vi "Acoustic Functional Test.vi"(0 "TSM context":T2, 5 "Limits File Path":path, 7 "Write to Limit File?":bool) -> (4 "Results":T1[](array[typedef]) {"Site Num" format="Site %#_g"}, 15 "error out":errorcluster)   [LabVIEW 2020]
doc: "Performs Functional test by sweeping over various frequency logarithmically over a single amplitude and getting the equivalent dB SPL. This Obtained dB SPL is compared with Limits files to validate \"In Range?\" functionality."
uses:
  <vilib>/NI_TestStand_SemiconductorModule/NI_TestStand_Semiconductor_Module.lvlibp/PinMap/General/SemiconductorModuleContext.ctl
  SubVIs/Site Info.ctl
  Common/Utility/Calibration Sweep/Sweep Parameters.ctl
  Limits File APIs/Plot Data.ctl
  <vilib>/NI_TestStand_SemiconductorModule/NI_TestStand_Semiconductor_Module.lvlibp
panel:
  in  "Exit":bool
  out "dBSPL Frequency Graph":cluster{"Frequency(Hz)":dbl[], "dB SPL":dbl[]}[](graph)
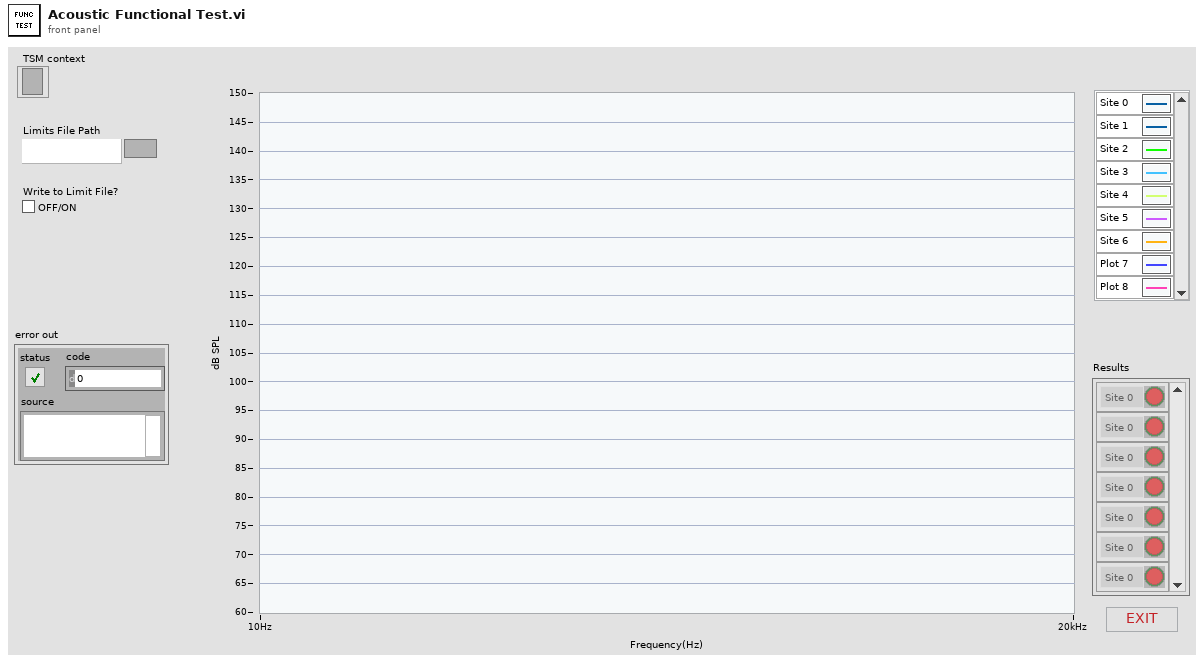
[diagram p1: front panel]
types:
  T1 = typedef "Site Info.ctl" = cluster{"Site Num":i32, "In Range?":bool}
  T2 = typedef "NI_TestStand_Semiconductor_Module.lvlibp/SemiconductorModuleContext.ctl" = refnum<k7>
  T3 = typedef "Sweep Parameters.ctl" = cluster{"Start":dbl, "End":dbl, "Samples":i32}
  T4 = typedef "Plot Data.ctl" = cluster{"Frequency(Hz)":dbl[], "dB SPL":dbl[]}
  T5 = cluster{"TSM context":T2, "Site Numbers":i32[], "Limits File Path":path, "Speaker Samp Rate (Hz)":dbl, "Ref Mic Samp Rate (Hz)":dbl, "Amplitude (V)":dbl, "Coarse Freq Sweep (Hz)":T3, "Fine Freq Sweep (Hz)":T3, "Positive Limit Plot":T4, "Negative Limit Plot":T4, "Graph Data":T4[], "Graph Ref":refnum<vi>, "Write Limit File?":bool, "Per-Site In Range?":T1[]}
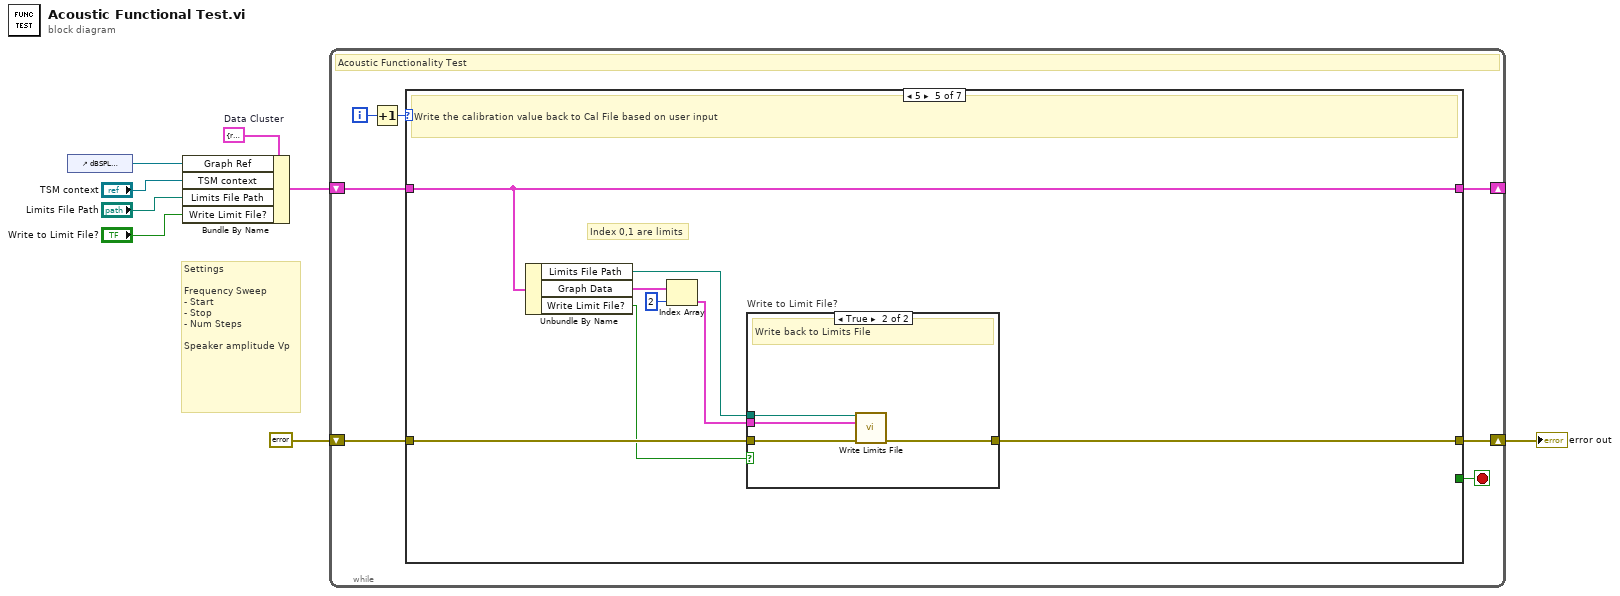
[diagram p0: block diagram]
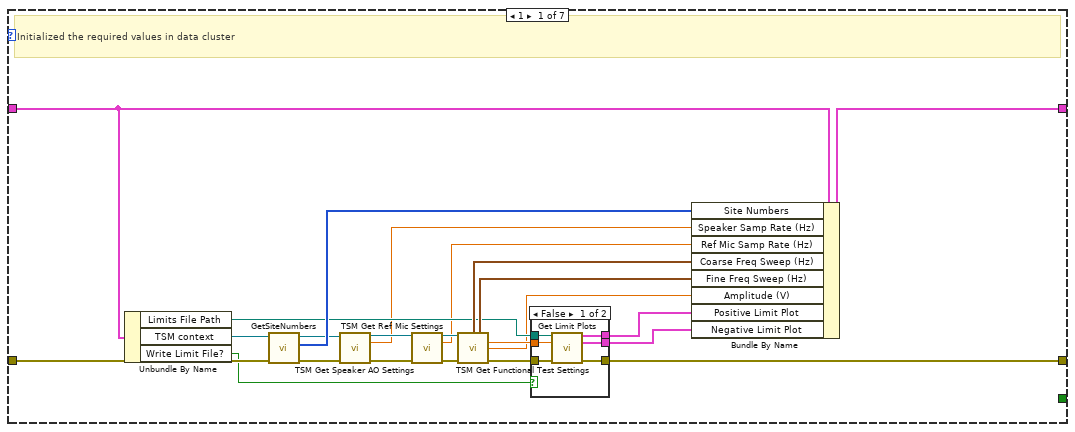
[diagram p2: hidden frame]
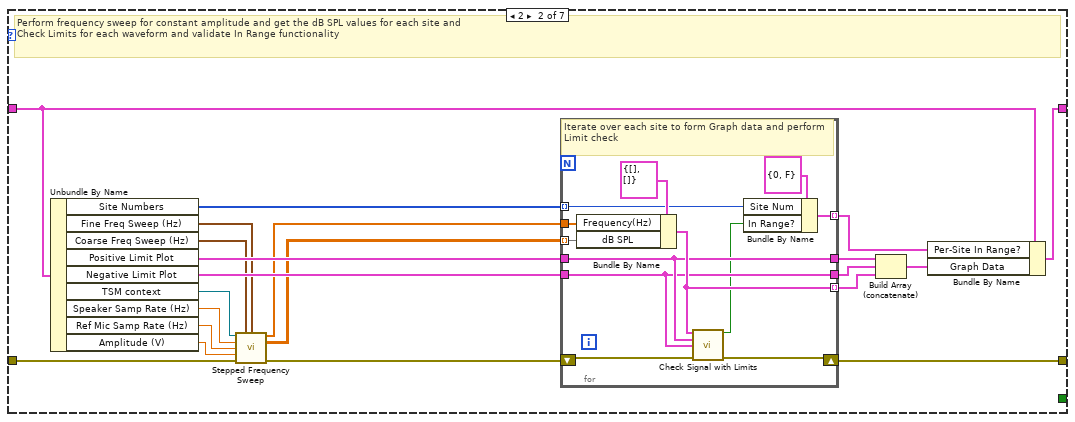
[diagram p4: hidden frame]
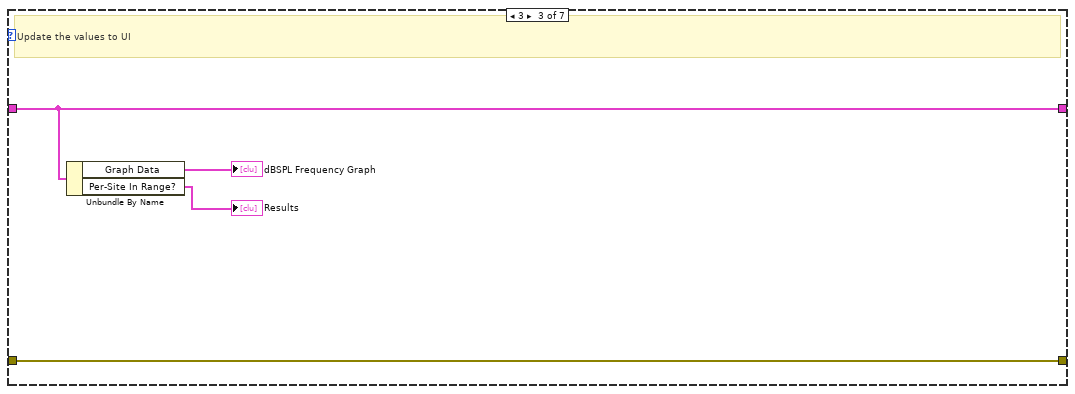
[diagram p5: hidden frame]
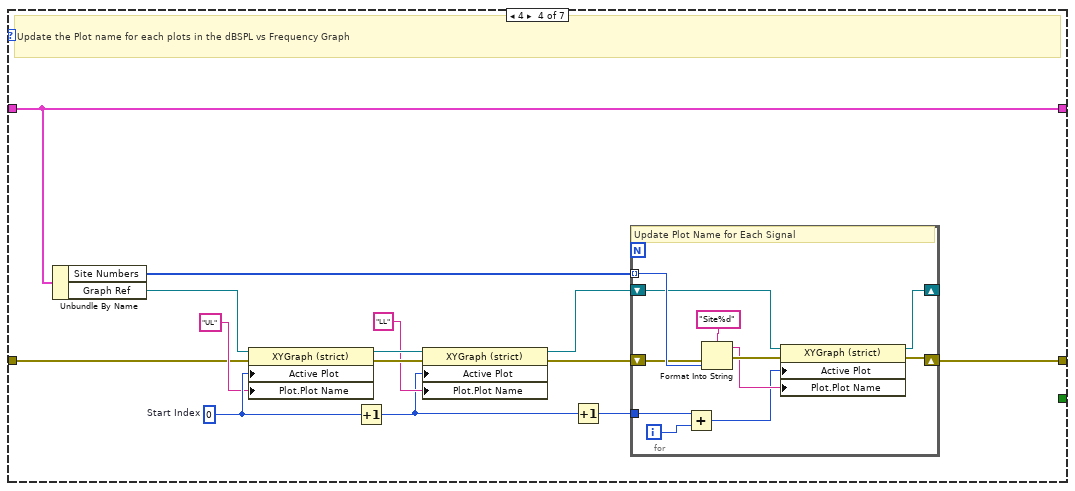
[diagram p6: hidden frame]
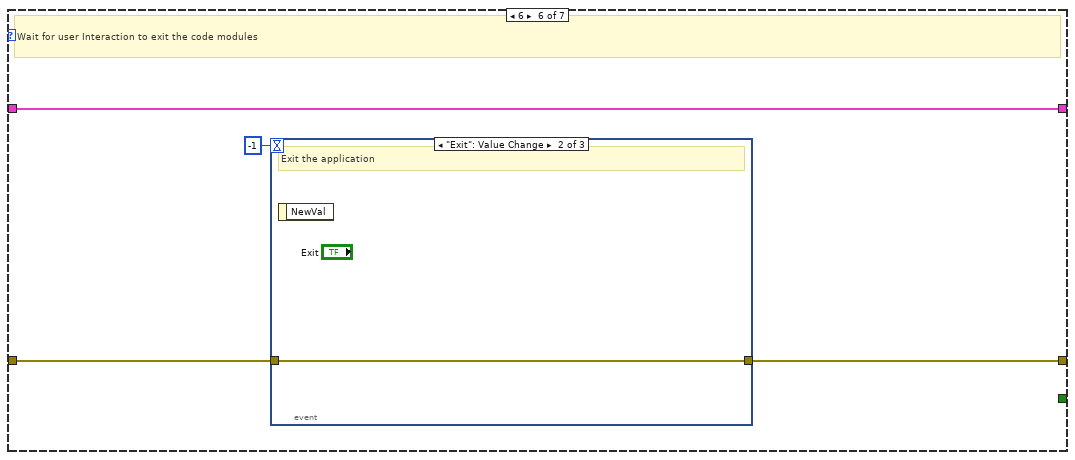
[diagram p8: hidden frame]
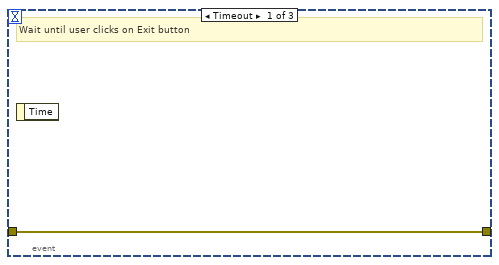
[diagram p9: hidden frame]
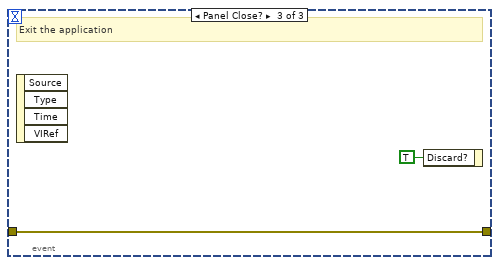
[diagram p10: hidden frame]
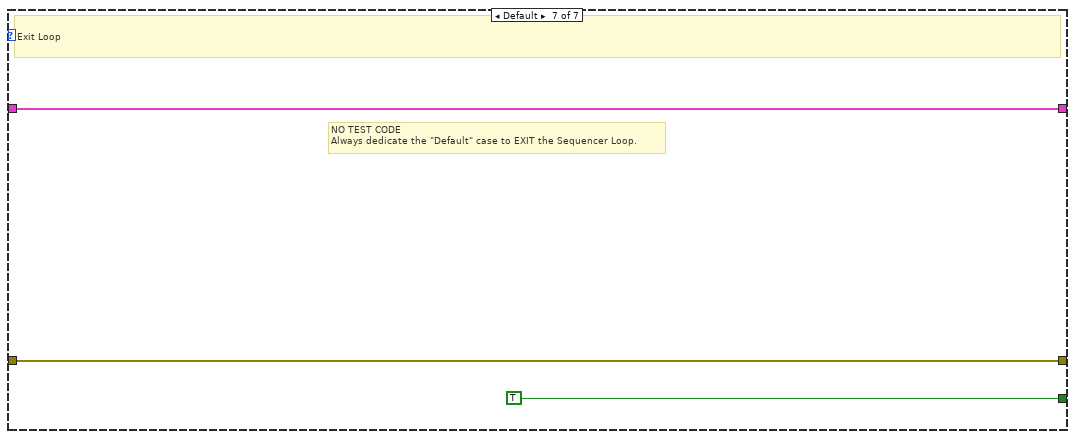
[diagram p11: hidden frame]
diagram:
  w6 = T5 {"TSM context"=refnum, "Site Numbers"=[], "Limits File Path"=path "", "Speaker Samp Rate (Hz)"=0.0, "Ref Mic Samp Rate (Hz)"=0.0, "Amplitude (V)"=0.0, "Coarse Freq Sweep (Hz)"={"Start"=0.0, "End"=0.0, "Samples"=0}, "Fine Freq Sweep (Hz)"={"Start"=0.0, "End"=0.0, "Samples"=0}, "Positive Limit Plot"={"Frequency(Hz)"=[], "dB SPL"=[]}, "Negative Limit Plot"={"Frequency(Hz)"=[], "dB SPL"=[]}, "Graph Data"=[], "Graph Ref"=refnum, "Write Limit File?"=FALSE, "Per-Site In Range?"=[]}  # Data Cluster
  # "Settings\n\nFrequency Sweep\n- Start\n- Stop\n- Num Steps\n\nSpeaker amplitude Vp"
  n1 = control-ref of="dBSPL Frequency Graph"() -> (w3:refnum<vi>)
  n2 = Bundle By Name(cluster=w6, "Graph Ref"=w3, "TSM context"="TSM context", "Limits File Path"="Limits File Path", "Write Limit File?"="Write to Limit File?") -> (w5:T5)
  n3 = while {
    shift-right: [w13] -> w8
    shift-left: errorcluster {"status"=FALSE, "code"=0, "source"=""} ("error in") -> [w14]
    shift-right: [w9] -> _
    shift-left: w5 -> [w10]
    i -> [w15]
    stop <- w11 stop-if-true
    # "Acoustic Functionality Test"
    n4 = Increment(x=w15) -> (x+1=w12:i32)
    n5 = case shown="5" w12 {
      tunnel: [w28 w63 w82 w83 w110 w122 w130] -> w13
      tunnel: w14 -> [w38 w57 w82 w89 w111 w123 w130]
      tunnel: [_ _ _ _ _ _ TRUE] -> w11
      tunnel: w10 -> [w35 w66 w81 w96 w115 w124 w129]
      tunnel: [w37 w62 w81 w96 w115 w124 w129] -> w9
      frame 1 {
        # "Initialized the required values in data cluster"
        n6 = Unbundle By Name(w35) -> ("Limits File Path"=w29:path, "TSM context"=w34:T2, "Write Limit File?"=w17:bool)
        n7 = call <vilib>:"GetSiteNumbers.vi"("error in (no error)"=w38, "Semiconductor Module Context"=w34) -> ("error out"=w23:errorcluster, "Site Numbers"=w36:i32[], "Semiconductor Module Context Out"=w22:T2)  [unwired: 6 in, 1 out]
        n8 = call "TSM Get Speaker AO Settings.vi"("TSM context"=w22, "error in (no error)"=w23) -> ("TSM context Out"=w21:T2, "Sampling Rate (Hz)"=w19:dbl, "error out"=w18:errorcluster)  [unwired: 9 in, 2 out]
        n9 = call "TSM Get Ref Mic Settings.vi"("TSM context"=w21, "error in (no error)"=w18) -> ("TSM context Out"=w24:T2, "Sampling Rate (Hz)"=w20:dbl, "error out"=w25:errorcluster)  [unwired: 8 in, 3 out]
        n10 = call "TSM Get Functional Test Settings.vi"("TSM context"=w24, "error in (no error)"=w25) -> ("Coarse Freq Sweep (Hz)"=w33:T3, "Fine Freq Sweep (Hz)"=w32:T3, "Limit (dB SPL)"=w30:dbl, "Speaker Amplitude (V)"=w16:dbl, "error out"=w31:errorcluster)  [unwired: 8 in, 1 out]
        n11 = case shown="False" w17 {
          tunnel: w31 -> [w44 w45]
          tunnel: w30 -> [w43 _]
          tunnel: w29 -> [w42 _]
          tunnel: [w41 w45] -> w28
          tunnel: [w40 _] -> w27
          tunnel: [w39 _] -> w26
          frame False {
            n12 = call "Get Limit Plots.vi"("Limits File Path"=w42, "Limit Range (dB SPL)"=w43, "error in (no error)"=w44) -> ("Positive Limit Plot"=w40:T4, "Negative Limit Plot"=w39:T4, "error out"=w41:errorcluster)  [unwired: 10 in]
          }
          frame True {
          }
        }
        n13 = Bundle By Name(cluster=w35, "Site Numbers"=w36, "Speaker Samp Rate (Hz)"=w19, "Ref Mic Samp Rate (Hz)"=w20, "Coarse Freq Sweep (Hz)"=w33, "Fine Freq Sweep (Hz)"=w32, "Amplitude (V)"=w16, "Positive Limit Plot"=w27, "Negative Limit Plot"=w26) -> (w37:T5)
      }
      frame 2 {
        # "Perform frequency sweep for constant amplitude and get the dB SPL values for each site and\nCheck Limits for each waveform and validate In Range functionality"
        n14 = Unbundle By Name(w66) -> ("Site Numbers"=w49:i32[], "Fine Freq Sweep (Hz)"=w54:T3, "Coarse Freq Sweep (Hz)"=w55:T3, "Positive Limit Plot"=w65:T4, "Negative Limit Plot"=w64:T4, "TSM context"=w53:T2, "Speaker Samp Rate (Hz)"=w52:dbl, "Ref Mic Samp Rate (Hz)"=w47:dbl, "Amplitude (V)"=w46:dbl)
        n15 = call "Stepped Frequency Sweep.vi"("Semiconductor Module Context"=w53, "Coarse Frequency Sweep (Hz)"=w55, "Fine Frequency Sweep (Hz)"=w54, "Speaker Sampling Rate (Hz)"=w52, "Ref Mic Sampling Rate (Hz)"=w47, "Amplitude (V)"=w46, "error in (no error)"=w57) -> ("Frequency (Hz)"=w51:dbl[], "Per-Site Per-Frequency dbSPL"=w50:dbl[][], "error out"=w56:errorcluster)  [unwired: 6 in]
        n16 = for {
          tunnel: [w73] -> w58 mode=indexing
          tunnel: w51 -> [w78]
          tunnel: w50 -> [w77] mode=indexing
          tunnel: w65 -> [w72]
          shift-right: [w74] -> w63
          shift-left: w56 -> [w75]
          tunnel: w64 -> [w71]
          tunnel: [w72] -> w61
          tunnel: [w71] -> w60
          tunnel: w49 -> [w69] mode=indexing
          tunnel: [w67] -> w48 mode=indexing
          # "Iterate over each site to form Graph data and perform Limit check"
          n17 = Bundle By Name(cluster=T4 {"Frequency(Hz)"=[], "dB SPL"=[]} ("Plot Data"), "Frequency(Hz)"=w78, "dB SPL"=w77) -> (w73:T4)
          n18 = call "Check Signal with Limits.vi"("Signal"=w73, "Positive Limit"=w72, "Negative Limit"=w71, "error in (no error)"=w75) -> ("In Range?"=w68:bool, "error out"=w74:errorcluster)  [unwired: 10 in]
          n19 = Bundle By Name(cluster=T1 {"Site Num"=0, "In Range?"=FALSE} ("Site Info"), "Site Num"=w69, "In Range?"=w68) -> (w67:T1)
        }
        n20 = Build Array (concatenate)(w61, w60, w58) -> (w59:T4[])
        n21 = Bundle By Name(cluster=w66, "Per-Site In Range?"=w48, "Graph Data"=w59) -> (w62:T5)
      }
      frame 3 {
        # "Update the values to UI"
        n22 = Unbundle By Name(w81) -> ("Graph Data"=→"dBSPL Frequency Graph":T4[], "Per-Site In Range?"=→"Results":T1[])
      }
      frame 4 {
        w94 = 0  # Start Index
        # "Update the Plot name for each plots in the dBSPL vs Frequency Graph"
        n23 = Unbundle By Name(w96) -> ("Site Numbers"=w95:i32[], "Graph Ref"=w87:refnum<vi>)
        n24 = property on="Property Node" class="XYGraph (strict)"(reference=w87, error in=w89, "Active Plot"=w94, "Plot.Plot Name"="UL" ("format string")) -> (reference out=w92:refnum<vi>, error out=w93:errorcluster)
        n25 = Increment(x=w94) -> (x+1=w85:i32)
        n26 = property on="Property Node" class="XYGraph (strict)"(reference=w92, error in=w93, "Active Plot"=w85, "Plot.Plot Name"="LL" ("format string")) -> (reference out=w86:refnum<vi>, error out=w88:errorcluster)
        n27 = Increment(x=w85) -> (x+1=w84:i32)
        n28 = for {
          shift-right: [w104] -> w83
          shift-left: w88 -> [w102]
          tunnel: w95 -> [w103] mode=indexing
          shift-right: [w100] -> _
          shift-left: w86 -> [w101]
          tunnel: w84 -> [w99]
          i -> [w98]
          # "Update Plot Name for Each Signal"
          n29 = Add(x=w99, y=w98) -> (x+y=w97:i32)
          n30 = Format Into String(format string="Site%d", error in=w102, w103) -> (resulting string=w105:string, error out=w106:errorcluster)  [unwired: 1 in]
          n31 = property on="Property Node" class="XYGraph (strict)"(reference=w101, error in=w106, "Active Plot"=w97, "Plot.Plot Name"=w105) -> (reference out=w100:refnum<vi>, error out=w104:errorcluster)
        }
      }
      frame 5 {
        # "Index 0,1 are limits"
        # "Write the calibration value back to Cal File based on user input"
        n32 = Unbundle By Name(w115) -> ("Limits File Path"=w113:path, "Graph Data"=w114:T4[], "Write Limit File?"=w109:bool)
        n33 = Index Array(array=w114, index=2) -> (element=w112:T4)
        n34 = case "Write to Limit File?" shown="True" w109 {
          tunnel: w113 -> [_ w120]
          tunnel: w112 -> [_ w119]
          tunnel: w111 -> [w116 w118]
          tunnel: [w116 w117] -> w110
          frame False {
            # "Skip writing to File"
          }
          frame True {
            # "Write back to Limits File"
            n35 = call "Write Limits File.vi"("Limits File Path"=w120, "Limit Data"=w119, "error in (no error)"=w118) -> ("error out"=w117:errorcluster)  [unwired: 12 in]
          }
        }
      }
      frame 6 {
        # "Wait for user Interaction to exit the code modules"
        n36 = event shown="[1] \"Exit\": Value Change" {
          selector: _ -> [_ _ _]
          dyn-events: _ -> [_ _ _]
          timeout: -1 -> [_ _ _]
          tunnel: w123 -> [w125 w126 w127]
          tunnel: [w125 w126 w127] -> w122
          event Timeout {
            # "Wait until user clicks on Exit button"
            n37 = event-data() -> ()  [unwired: 1 in, 1 out]
          }
          event "Exit": Value Change {
            # "Exit the application"
            n38 = event-data() -> ()  [unwired: 1 in, 1 out]
          }
          event Panel Close? {
            # "Exit the application"
            n39 = event-data() -> ()  [unwired: 1 in, 4 out]
            n40 = event-data("Discard?"=TRUE) -> ()  [unwired: 1 in, 1 out]
          }
        }
      }
      frame Default {
        # "NO TEST CODE\nAlways dedicate the \"Default\" case to EXIT the Sequencer Loop."
        # "Exit Loop"
      }
    }
  }
  "error out" <- w8
